vi "Configure GPIB.vi"(8 "error in":errorcluster, 11 "VISA Refnum in":refnum<visa-resource-name>) -> (0 "error out":errorcluster, 3 "VISA resource name out":refnum<visa-resource-name>)   [LabVIEW 2015, in "Yokogawa.lvclass"]
uses:
  Power Meter/Yokogawa/Yokogawa.lvclass
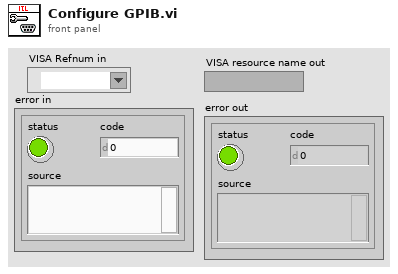
[diagram p1: front panel]
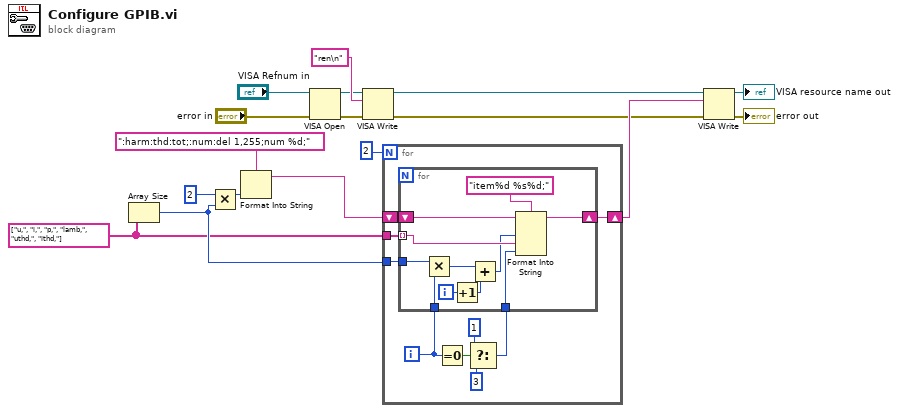
[diagram p0: block diagram]
diagram:
  w11 = string[] ["u,", "i,", "p,", "lamb,", "uthd,", "ithd,"]
  n1 = Array Size(array=w11) -> (size(s)=w14:i32)
  n2 = Multiply(x=2 ("y"), y=w14) -> (x*y=w16:i32)
  n3 = Format Into String(format string=":harm:thd:tot;:num:del 1,255;num %d;", w16) -> (resulting string=w13:string)  [unwired: 2 in, 1 out]
  n4 = VISA Open(error in (no error)="error in", VISA resource name="VISA Refnum in") -> (VISA resource name=w7:refnum<visa-resource-name>, error out=w8:errorcluster)  [unwired: 3 in]
  n5 = VISA Write(VISA resource name=w7, write buffer="ren\n", error in (no error)=w8) -> (VISA resource name out=w1:refnum<visa-resource-name>, error out=w6:errorcluster)  [unwired: 1 out]
  n6 = for {
    N: 2 -> [_]
    shift-right: [w24] -> w17
    shift-left: w13 -> [w26]
    tunnel: w11 -> [w25]
    tunnel: w14 -> [w23]
    i -> [w22]
    n7 = Equal To 0?(x=w22) -> (x = 0?=w21:bool)
    n8 = Select(t=1, s=w21, f=3) -> (s? t:f=w18:i32)
    n9 = for {
      shift-right: [w35] -> w24
      shift-left: w26 -> [w36]
      tunnel: w25 -> [w34] mode=indexing
      tunnel: w18 -> [w32]
      tunnel: w22 -> [w30]
      tunnel: w23 -> [w31]
      i -> [w33]
      n10 = Multiply(x=w31, y=w30) -> (x*y=w29:i32)
      n11 = Increment(x=w33) -> (x+1=w28:i32)
      n12 = Add(x=w29, y=w28) -> (x+y=w27:i32)
      n13 = Format Into String(format string="item%d %s%d;", initial string=w36, w27, w34, w32) -> (resulting string=w35:string)  [unwired: 1 in, 1 out]
    }
  }
  n14 = VISA Write(VISA resource name=w1, write buffer=w17, error in (no error)=w6) -> (VISA resource name out=→"VISA resource name out":refnum<visa-resource-name>, error out=→"error out":errorcluster)  [unwired: 1 out]
